vi "Amps Display.vi"(7 "String IN":string, 9 "Pump Current":dbl[](array[numeric]), 10 "Controller Current":dbl[](array[numeric]), 11 "Controller Type:":T1) -> (6 "String OUT":string)   [LabVIEW 2019]
uses:
  Type Defs/Controller Names.ctl
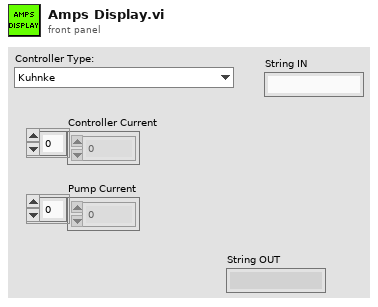
[diagram p1: front panel]
types:
  T1 = typedef "Controller Names.ctl" = enum16{"Kuhnke", "Helbako BLDC", "Conti", "Hella BLDC OL PWM", "Hella BLDC Turbine OL PWM", "Hella BLDC Pressure", "Helbako (old)", "TI PWM", "PSA", "Hella Gas", "Hella Diesel", "8 Comm", "10 Comm", "8 Comm Hella", "10 Comm Hella", "8 Comm Omron", "10 Comm Omron", "8 Comm Nissan", "10 Comm Nissan"}
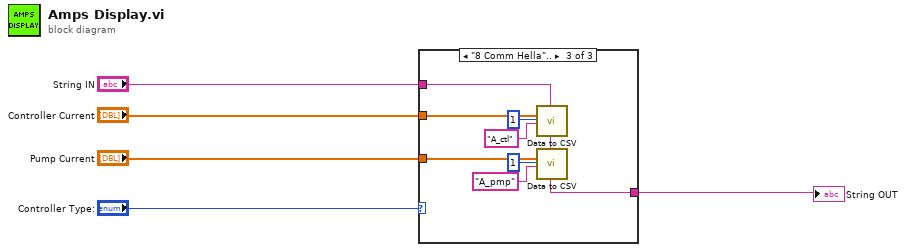
[diagram p0: block diagram]
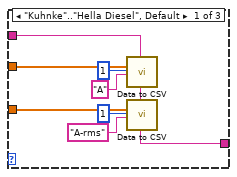
[diagram p2: hidden frame]
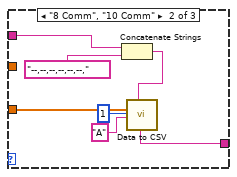
[diagram p3: hidden frame]
diagram:
  n1 = case shown="\"8 Comm Hella\".." "Controller Type:" {
    tunnel: "Pump Current" -> [w14 w21 w30]
    tunnel: "Controller Current" -> [w13 _ w29]
    tunnel: [w12 w20 w28] -> w3
    tunnel: "String IN" -> [w6 w17 w22]
    frame "Kuhnke".."Hella Diesel", Default {
      n2 = call "Data to CSV.vi"("Data Array"=w13, "Precision (0)"=i16 1, "Units"="A", "String IN"=w6) -> ("String OUT"=w11:string)  [unwired: 23 in]
      n3 = call "Data to CSV.vi"("Data Array"=w14, "Precision (0)"=i16 1, "Units"="A-rms", "String IN"=w11) -> ("String OUT"=w12:string)  [unwired: 23 in]
    }
    frame "8 Comm", "10 Comm" {
      n4 = Concatenate Strings(w17, "--,--,--,--,--,--," ("Units")) -> (w15:string)
      n5 = call "Data to CSV.vi"("Data Array"=w21, "Precision (0)"=i16 1, "Units"="A", "String IN"=w15) -> ("String OUT"=w20:string)  [unwired: 23 in]
    }
    frame "8 Comm Hella".. {
      n6 = call "Data to CSV.vi"("Data Array"=w29, "Precision (0)"=i16 1, "Units"="A_ctl", "String IN"=w22) -> ("String OUT"=w27:string)  [unwired: 23 in]
      n7 = call "Data to CSV.vi"("Data Array"=w30, "Precision (0)"=i16 1, "Units"="A_pmp", "String IN"=w27) -> ("String OUT"=w28:string)  [unwired: 23 in]
    }
  }
  "String OUT" <- w3
